vi "_PC_RTFunc_AccessScript.vi"(7 "Function":enum16{"Write", "Read"}(ring)=enum."Read", 8 "error in (no error)":errorcluster, 9 "Var in":variant) -> (0 "error out":errorcluster, 1 "Var out":variant)   [LabVIEW 2018]
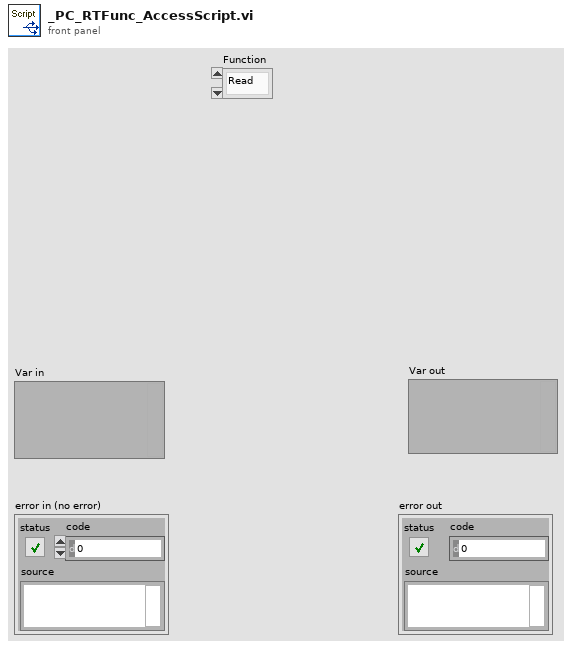
[diagram p1: front panel]
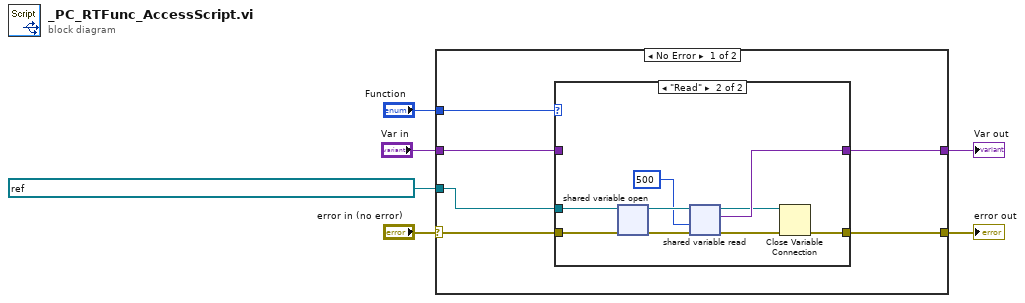
[diagram p0: block diagram]
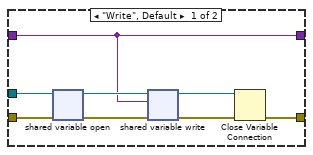
[diagram p2: hidden frame]
diagram:
  n1 = case shown="No Error" "error in (no error)" {
    selector: "error in (no error)" -> [w9 w31]
    tunnel: refnum<k21> "ni.var.psp://NI-sbRIO/_RT_CtrlLoop_WfmData_Variable/Wfm_Script" ("shared variable refnum in") -> [w12 _]
    tunnel: "Function" -> [w11 _]
    tunnel: [w10 w31] -> w2
    tunnel: [w7 w30] -> w1
    tunnel: "Var in" -> [w8 w30]
    frame No Error {
      n2 = case shown="\"Read\"" w11 {
        tunnel: w12 -> [w20 w29]
        tunnel: [w14 w28] -> w10
        tunnel: w9 -> [w19 w27]
        tunnel: [w13 w25] -> w7
        tunnel: w8 -> [w13 _]
        frame "Write", Default {
          n3 = shared-variable-open(w20, w19) -> (w18:refnum<k21>, w17:errorcluster)
          n4 = shared-variable-write(w18, w17, w13) -> (w16:refnum<k21>, w15:errorcluster)
          n5 = Close Variable Connection(8:w15, 11:w16) -> (0:w14:errorcluster)
        }
        frame "Read" {
          n6 = shared-variable-open(w29, w27) -> (w26:refnum<k21>, w23:errorcluster)
          n7 = shared-variable-read(w26, w23, 500 ("timeout ms")) -> (w24:refnum<k21>, w22:errorcluster, w25:variant)  [unwired: 1 out]
          n8 = Close Variable Connection(8:w22, 11:w24) -> (0:w28:errorcluster)
        }
      }
    }
    frame Error {
    }
  }
  "error out" <- w2
  "Var out" <- w1
